vi "WFComposeCanD.vi"(8 "error in (no error)":errorcluster, 10 "Cluster":T1={"Del (s)"=0.0, "Int (s)"=0.0, "N"=1} {"Int (s)" min=0.0 format="%#_4g"; "Del (s)" min=0.0 format="%#_4f"}, 11 "Waveform In":digitalwaveform(waveform)={"t0"=timestamp(0 s since 1904-01-01), "dt"=1.0, "Y"={"transitions"=[], "data"=[]}}) -> (0 "error out":errorcluster, 3 "ComposeCan":bool)   [LabVIEW 2013]
uses:
  WFRepetitions.ctl
  <vilib>/Utility/error.llb/DialogType.ctl
  <vilib>/Waveform/DWDTOps.llb/DWDT Waveform Duration.vi
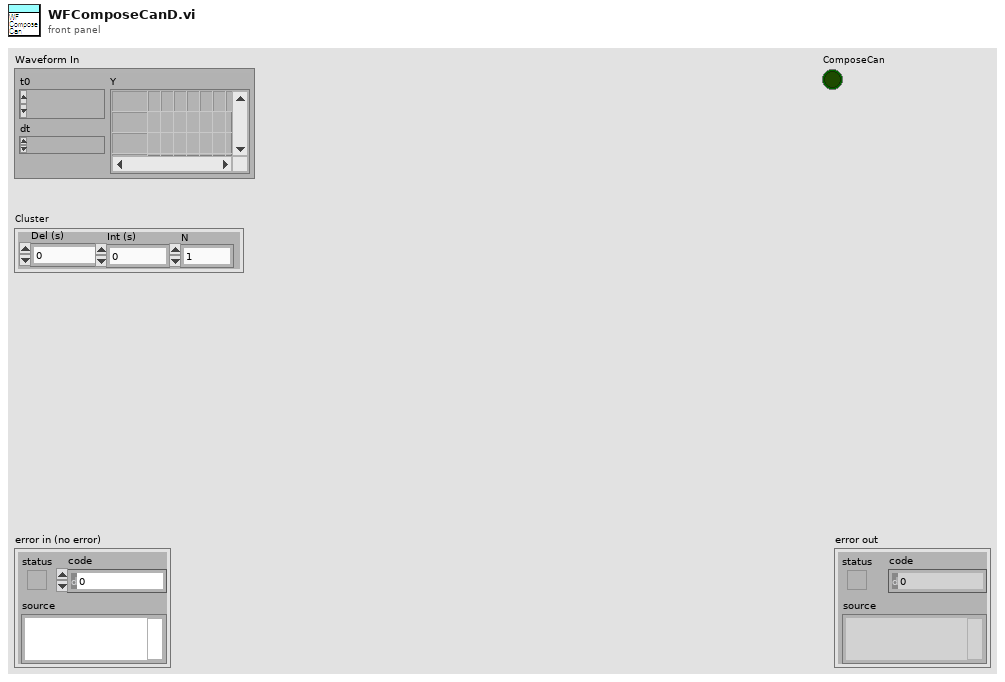
[diagram p1: front panel]
types:
  T1 = typedef "WFRepetitions.ctl" = cluster{"Del (s)":dbl, "Int (s)":dbl, "N":i32}
  T2 = typedef "DialogType.ctl" = u16
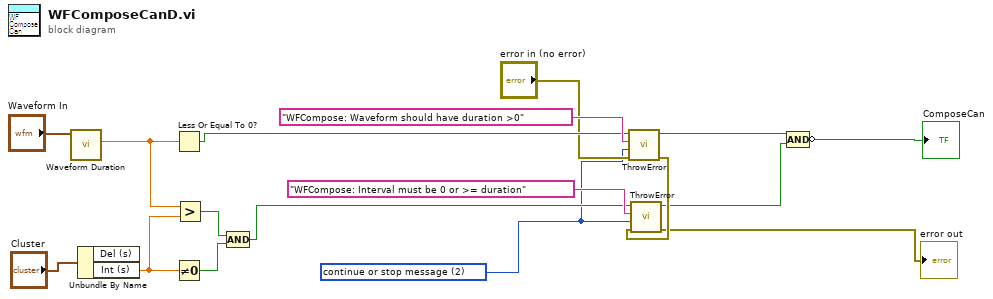
[diagram p0: block diagram]
diagram:
  w1 = T2 2 items=["no dialog", "OK message", "continue or stop message", "OK message + warnings", "continue/stop + warnings"] ("type of dialog (OK msg:1)")
  n1 = call-poly <vilib>:"Waveform Duration.vi"("waveform in"="Waveform In") -> ("duration"=w16:dbl)  [unwired: 8 in, 2 out]
  n2 = Unbundle By Name("Cluster") -> ("Int (s)"=w13:dbl)  [unwired: 1 out]
  n3 = Less Or Equal To 0?(x=w16) -> (x <= 0?=w11:bool)
  n4 = Not Equal To 0?(x=w13) -> (x != 0?=w15:bool)
  n5 = Greater?(x=w16, y=w13) -> (0:w8:bool)
  n6 = Compound Arithmetic op=AND(w8, w15) -> (w7:bool)
  n7 = call "ThrowError.vi"("error in (no error)"="error in (no error)", "type of dialog (OK msg:1)"=w1, "Error Message"="WFCompose: Waveform should have duration >0", "Error Input"=w11) -> ("error out"=w5:errorcluster, "Error Input Passthrough"=w10:bool)  [unwired: 6 in]
  n8 = call "ThrowError.vi"("error in (no error)"=w5, "type of dialog (OK msg:1)"=w1, "Error Message"="WFCompose: Interval must be 0 or >= duration", "Error Input"=w7) -> ("error out"=→"error out":errorcluster, "Error Input Passthrough"=w3:bool)  [unwired: 6 in]
  n9 = Compound Arithmetic op=AND(w10, w3) -> (invert →"ComposeCan":bool)
